vi "Make Default FFmeter settings.vi"() -> (3 "FFmeter settings":T1={"AC Source"={"AC Source type"=enum."Agilent 331xxA to 332xxA", "awg lib session"={"type"=enum."Agilent 331xxA to 332xxA", "VISA"="", "enable 10MHz ref"=FALSE, "cmi ckd2"={"VISA"="", "clock source"=enum."Auto", "manual ref clk"=FALSE, "ref clock [Hz]"=0.0, "div mode"=enum."Set divisor directly"}, "cmi sync v3"={"VISA"="", "baud rate [bd/s]"=115200, "source"=enum."Auto", "hv range"=enum."1kV", "fsrc is fixed"=FALSE, "fsrc [Hz]"=10000000.0, "freq integ [s]"=1.0, "freq filter"=5, "trig level"=enum."TTL 5V", "chn1 mode"=enum."Source divider", "chn1 level"=enum."Positive 5V", "chn2 mode"=enum."Source divider", "chn2 level"=enum."Positive 5V", "chn2 div"=1, "chn3 mode"=enum."Chn 1 Active", "chn3 level"=enum."Positive 5V", "chn1 div entry"=enum."Calculate nearest divisor from measured fx", "chn1 dev limit [%]"=1.0, "chn1 check dev"=FALSE}, "trigger"={"source"=enum."Immediate", "level [V]"=0.0, "coupling"=enum."DC", "slope"=enum."POS"}, "HMF2500 cfg"={"Baud Rate"=9600, "Parity"=0, "Data Bits"=8, "Flow Control"=4}}, "DAQmx Device Name"="PXI2Slot6"}, "TWM pipe"="\\\\.\\pipe\\TWM:server", "Measurement status ref"=refnum, "TWM Status ref"=refnum, "Abort ref"=refnum, "AC Source  status ref"=refnum, "DC meter"={"DC meter type"=enum."H/A/K 3458", "DC meter VISA"="", "NPLC"=10.0}, "Measurement properties"={"Measurement frequencies (Hz)"=[1000.0], "Sampling frequency (Hz)"=500000.0, "Signal amplitude (V)"=4.5, "AC-DC settle time (s)"=20.0, "Record length (multiples of period)"=[1000.0, 10000.0, 1000.0], "Measurement template file"=path "", "Row of START keyword"=1, "Row of STOP keyword"=0}} {"Measurement properties"."Record length (multiples of period)" format="%#_3p"; "Measurement properties"."Sampling frequency (Hz)" format="%#_3p"; "Measurement properties"."Measurement frequencies (Hz)" format="%#_3p"; "AC Source"."awg lib session"."HMF2500 cfg"."Flow Control" items=["None", "XON/XOFF", "RTS/CTS", "XON/XOFF & RTS/CTS", "DTR/DSR", "XON/XOFF & DTR/DSR"]; "AC Source"."awg lib session"."HMF2500 cfg"."Data Bits" items=["7"=7, "8"=8]; "AC Source"."awg lib session"."HMF2500 cfg"."Parity" items=["None", "Odd", "Even", "Mark", "Space"]; "AC Source"."awg lib session"."HMF2500 cfg"."Baud Rate" items=["300"=300, "600"=600, "1200"=1200, "2400"=2400, "4800"=4800, "9600"=9600, "19200"=19200]; "AC Source"."awg lib session"."cmi sync v3"."chn2 div" min=1 max=100000000 step=1; "AC Source"."awg lib session"."cmi sync v3"."fsrc [Hz]" format="%_8p"})   [LabVIEW 2020]
doc: "Returns QPS set to default values."
uses:
  GUI/Type definitions/FFmeter settings.ctl
  General AC source/Type definitions/AC Source.ctl
  General AC source/Type definitions/AC Source type.ctl
  external libraries/AWG/AWG Session.ctl
  external libraries/AWG/AWG Type.ctl
  external libraries/AWG/CMI Clock Divider v2/CMI ckd2 Session.ctl
  external libraries/AWG/CMI Clock Divider v2/CMI ckd2 Source Mode.ctl
  external libraries/AWG/CMI Clock Divider v2/CMI ckd2 Divisor Mode.ctl
  external libraries/AWG/CMI Sync V3/CMI Sync V3 session.ctl
  external libraries/AWG/CMI Sync V3/Configure/CMI Sync V3 Reference Clock Source.ctl
  external libraries/AWG/CMI Sync V3/Configure/CMI Sync V3 HV input Range.ctl
  external libraries/AWG/CMI Sync V3/Configure/CMI Sync V3 Trigger Input Level.ctl
  external libraries/AWG/CMI Sync V3/Configure/CMI Sync V3 Channel 1 Mode.ctl
  external libraries/AWG/CMI Sync V3/Configure/CMI Sync V3 Channel Output Levels.ctl
  external libraries/AWG/CMI Sync V3/Configure/CMI Sync V3 Channel 2 Mode.ctl
  external libraries/AWG/CMI Sync V3/Configure/CMI Sync V3 Channel 3 Mode.ctl
  external libraries/AWG/CMI Sync V3/Configure/CMI Sync V3 Channel 1 Divisor Entry Mode.ctl
  external libraries/externals needed for AWG/ADC Trig Config.ctl
  external libraries/externals needed for AWG/ADC Trig Mode Source.ctl
  external libraries/externals needed for AWG/ADC Trig Coupling.ctl
  external libraries/externals needed for AWG/ADC Trig Slope.ctl
  external libraries/AWG/RaS HMF2500/HMF2500 Config.ctl
  General DC meter/Type definitions/DC meter.ctl
  General DC meter/Type definitions/DC meter type.ctl
  Measurement/Type definitions/Measuement properties.ctl
  external libraries/AWG/AWG.lvlib
  external libraries/AWG/CMI Sync V3/CMI Sync Unit V3.lvlib
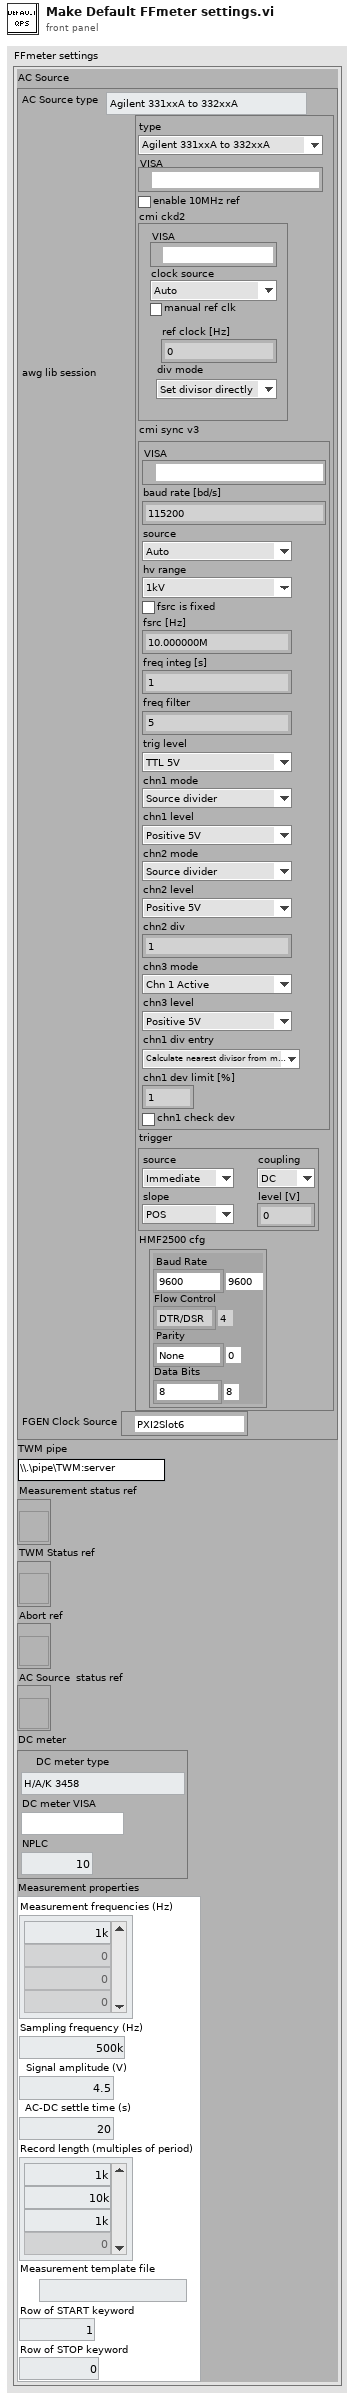
[diagram p1: front panel]
types:
  T1 = typedef "FFmeter settings.ctl" = cluster{"AC Source":T2, "TWM pipe":string, "Measurement status ref":refnum<vi>, "TWM Status ref":refnum<vi>, "Abort ref":refnum<vi>, "AC Source  status ref":refnum<vi>, "DC meter":T23, "Measurement properties":T25}
  T2 = typedef "AC Source.ctl" = cluster{"AC Source type":T3, "awg lib session":T4, "DAQmx Device Name":tag}
  T3 = typedef "AC Source type.ctl" = enum16{"Agilent 331xxA to 332xxA", "Agilent 335xxA to 336xxA", "Tektronix AFG3101C", "R&S HMF25xx", "CMI Clock Divider v2", "CMI Sync Unit V3", "NI DAQ", "Fluke 5XXX calibrator", "dummy"}
  T4 = typedef "AWG.lvlib/AWG Session.ctl" = cluster{"type":T5, "VISA":refnum<visa-resource-name>, "enable 10MHz ref":bool, "cmi ckd2":T6, "cmi sync v3":T9, "trigger":T18, "HMF2500 cfg":T22}
  T5 = typedef "AWG.lvlib/AWG Type.ctl" = enum16{"Agilent 331xxA to 332xxA", "Agilent 335xxA to 336xxA", "Tektronix AFG3101C", "R&S HMF25xx", "CMI Clock Divider v2", "CMI Sync Unit V3", "dummy"}
  T6 = typedef "AWG.lvlib/CMI ckd2 Session.ctl" = cluster{"VISA":refnum<visa-resource-name>, "clock source":T7, "manual ref clk":bool, "ref clock [Hz]":dbl, "div mode":T8}
  T7 = typedef "AWG.lvlib/CMI ckd2 Source Mode.ctl" = enum16{"Auto", "LF clock", "HF clock", "Internal"}
  T8 = typedef "AWG.lvlib/CMI ckd2 Divisor Mode.ctl" = enum16{"Set divisor directly", "Set divisor by frequency"}
  T9 = typedef "AWG.lvlib/CMI Sync Unit V3.lvlib/CMI Sync V3 session.ctl" = cluster{"VISA":refnum<visa-resource-name>, "baud rate [bd/s]":i32, "source":T10, "hv range":T11, "fsrc is fixed":bool, "fsrc [Hz]":dbl, "freq integ [s]":dbl, "freq filter":i32, "trig level":T12, "chn1 mode":T13, "chn1 level":T14, "chn2 mode":T15, "chn2 level":T14, "chn2 div":i32, "chn3 mode":T16, "chn3 level":T14, "chn1 div entry":T17, "chn1 dev limit [%]":dbl, "chn1 check dev":bool}
  T10 = typedef "AWG.lvlib/CMI Sync Unit V3.lvlib/CMI Sync V3 Reference Clock Source.ctl" = enum16{"Auto", "Internal", "Logic", "Sine", "HV"}
  T11 = typedef "AWG.lvlib/CMI Sync Unit V3.lvlib/CMI Sync V3 HV input Range.ctl" = enum16{"10V", "60V", "250V", "1kV"}
  T12 = typedef "AWG.lvlib/CMI Sync Unit V3.lvlib/CMI Sync V3 Trigger Input Level.ctl" = enum16{"LVCMOS 3V3", "TTL 5V"}
  T13 = typedef "AWG.lvlib/CMI Sync Unit V3.lvlib/CMI Sync V3 Channel 1 Mode.ctl" = enum16{"Source divider", "DDS absolute", "DDS ratio", "DDS ratio M/N"}
  T14 = typedef "AWG.lvlib/CMI Sync Unit V3.lvlib/CMI Sync V3 Channel Output Levels.ctl" = enum16{"Positive 3V3", "Negative 3V3", "Positive 5V", "Negative 5V"}
  T15 = typedef "AWG.lvlib/CMI Sync Unit V3.lvlib/CMI Sync V3 Channel 2 Mode.ctl" = enum16{"Source divider", "Chn 1 divide"}
  T16 = typedef "AWG.lvlib/CMI Sync Unit V3.lvlib/CMI Sync V3 Channel 3 Mode.ctl" = enum16{"Chn 1 Active", "Chn 2 Active", "Chn 1 Trigger", "Chn 2 Trigger", "Gate", "PPS", "10MHz"}
  T17 = typedef "AWG.lvlib/CMI Sync Unit V3.lvlib/CMI Sync V3 Channel 1 Divisor Entry Mode.ctl" = enum16{"Set divisor directly", "Calculate nearest divisor from measured fx"}
  T18 = typedef "ADC Trig Config.ctl" = cluster{"source":T19, "level [V]":dbl, "coupling":T20, "slope":T21}
  T19 = typedef "ADC Trig Mode Source.ctl" = enum16{"Immediate", "External", "Level"}
  T20 = typedef "ADC Trig Coupling.ctl" = enum16{"DC", "AC"}
  T21 = typedef "ADC Trig Slope.ctl" = enum16{"POS", "NEG"}
  T22 = typedef "AWG.lvlib/HMF2500 Config.ctl" = cluster{"Baud Rate":u32, "Parity":u16, "Data Bits":u16, "Flow Control":u16}
  T23 = typedef "DC meter.ctl" = cluster{"DC meter type":T24, "DC meter VISA":refnum<visa-resource-name>, "NPLC":dbl}
  T24 = typedef "DC meter type.ctl" = enum16{"H/A/K 3458", "FLuke 8508A", "dummy"}
  T25 = typedef "Measuement properties.ctl" = cluster{"Measurement frequencies (Hz)":dbl[], "Sampling frequency (Hz)":dbl, "Signal amplitude (V)":dbl, "AC-DC settle time (s)":dbl, "Record length (multiples of period)":dbl[], "Measurement template file":path, "Row of START keyword":i32, "Row of STOP keyword":i32}
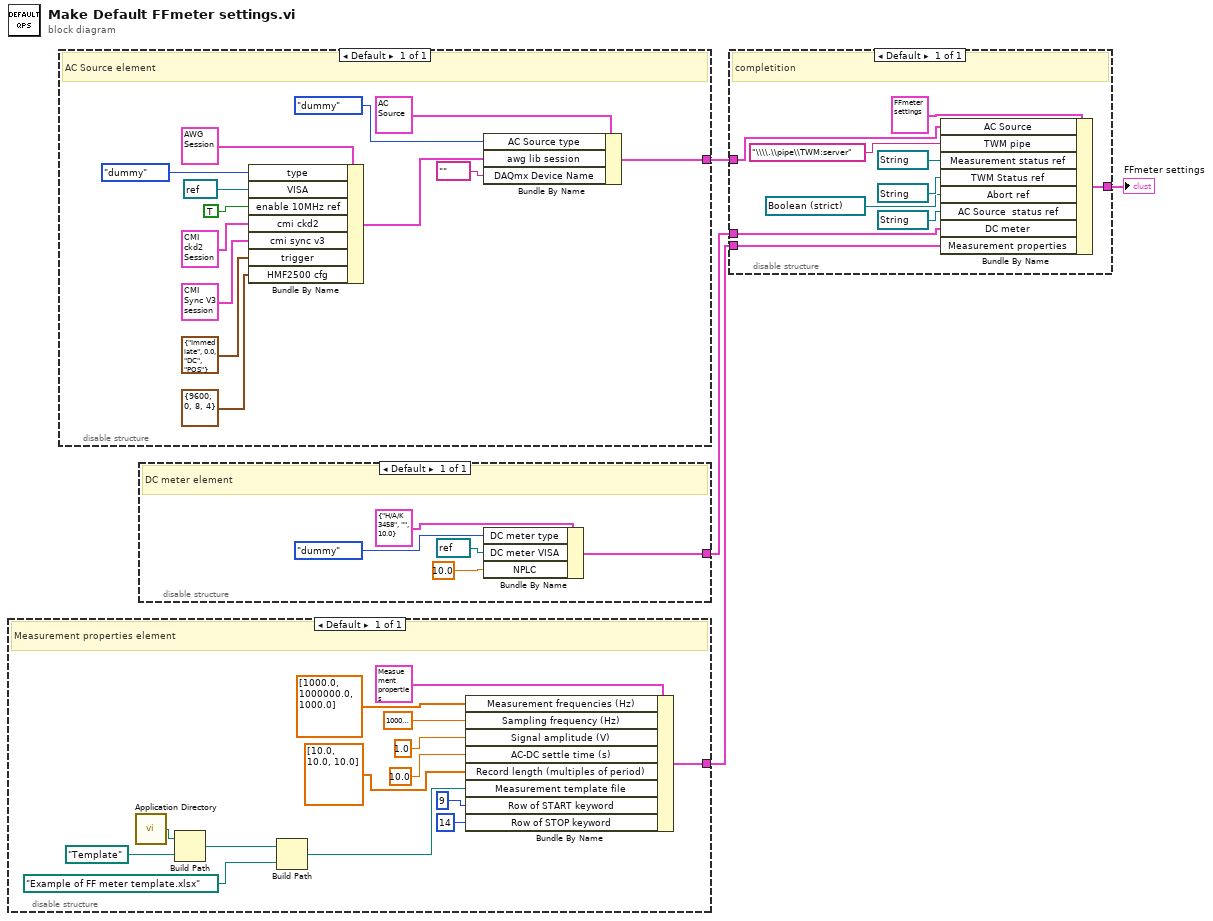
[diagram p0: block diagram]
diagram:
  n1 = disable-structure shown="Default" {
    disable-tunnel: [w17] -> w1
    frame Enabled {
      # "Measurement properties element"
      n2 = call <vilib>:"Application Directory.vi"() -> ("Application Directory"=w5:path)
      n3 = Build Path(base path=w5, name or relative path=path "Template") -> (appended path=w8:path)
      n4 = Build Path(base path=w8, name or relative path=path "Example of FF meter template.xlsx") -> (appended path=w6:path)
      n5 = Bundle By Name(cluster=T25 {"Measurement frequencies (Hz)"=[1000.0, 10000.0, 1000.0], "Sampling frequency (Hz)"=500000.0, "Signal amplitude (V)"=4.5, "AC-DC settle time (s)"=20.0, "Record length (multiples of period)"=[1000.0, 10000.0, 1000.0], "Measurement template file"=path "", "Row of START keyword"=0, "Row of STOP keyword"=0} ("Measurement properties"), "Measurement frequencies (Hz)"=dbl[] [1000.0, 1000000.0, 1000.0], "Sampling frequency (Hz)"=10000000.0, "Signal amplitude (V)"=1.0, "AC-DC settle time (s)"=10.0, "Record length (multiples of period)"=dbl[] [10.0, 10.0, 10.0], "Measurement template file"=w6, "Row of START keyword"=9, "Row of STOP keyword"=14) -> (w17:T25)
    }
  }
  n6 = disable-structure shown="Default" {
    disable-tunnel: [w22] -> w4
    frame Enabled {
      # "AC Source element"
      n7 = Bundle By Name(cluster=T4 {"type"=enum."Agilent 331xxA to 332xxA", "VISA"="", "enable 10MHz ref"=FALSE, "cmi ckd2"={"VISA"="", "clock source"=enum."Auto", "manual ref clk"=FALSE, "ref clock [Hz]"=0.0, "div mode"=enum."Set divisor directly"}, "cmi sync v3"={"VISA"="", "baud rate [bd/s]"=115200, "source"=enum."Auto", "hv range"=enum."1kV", "fsrc is fixed"=FALSE, "fsrc [Hz]"=10000000.0, "freq integ [s]"=1.0, "freq filter"=5, "trig level"=enum."TTL 5V", "chn1 mode"=enum."Source divider", "chn1 level"=enum."Positive 5V", "chn2 mode"=enum."Source divider", "chn2 level"=enum."Positive 5V", "chn2 div"=1, "chn3 mode"=enum."Chn 1 Active", "chn3 level"=enum."Positive 5V", "chn1 div entry"=enum."Calculate nearest divisor from measured fx", "chn1 dev limit [%]"=1.0, "chn1 check dev"=FALSE}, "trigger"={"source"=enum."Immediate", "level [V]"=0.0, "coupling"=enum."DC", "slope"=enum."POS"}, "HMF2500 cfg"={"Baud Rate"=9600, "Parity"=0, "Data Bits"=8, "Flow Control"=4}} ("awg session"), "type"=AWG_Type."dummy", "VISA"=refnum<visa-resource-name> refnum, "enable 10MHz ref"=TRUE, "cmi ckd2"=T6 {"VISA"="", "clock source"=enum."Auto", "manual ref clk"=FALSE, "ref clock [Hz]"=0.0, "div mode"=enum."Set divisor directly"}, "cmi sync v3"=T9 {"VISA"="", "baud rate [bd/s]"=115200, "source"=enum."Auto", "hv range"=enum."1kV", "fsrc is fixed"=FALSE, "fsrc [Hz]"=10000000.0, "freq integ [s]"=1.0, "freq filter"=5, "trig level"=enum."TTL 5V", "chn1 mode"=enum."Source divider", "chn1 level"=enum."Positive 5V", "chn2 mode"=enum."Source divider", "chn2 level"=enum."Positive 5V", "chn2 div"=1, "chn3 mode"=enum."Chn 1 Active", "chn3 level"=enum."Positive 5V", "chn1 div entry"=enum."Calculate nearest divisor from measured fx", "chn1 dev limit [%]"=1.0, "chn1 check dev"=FALSE}, "trigger"=T18 {"source"=enum."Immediate", "level [V]"=0.0, "coupling"=enum."DC", "slope"=enum."POS"}, "HMF2500 cfg"=T22 {"Baud Rate"=9600, "Parity"=0, "Data Bits"=8, "Flow Control"=4}) -> (w23:T4)
      n8 = Bundle By Name(cluster=T2 {"AC Source type"=enum."Agilent 331xxA to 332xxA", "awg lib session"={"type"=enum."Agilent 331xxA to 332xxA", "VISA"="", "enable 10MHz ref"=FALSE, "cmi ckd2"={"VISA"="", "clock source"=enum."Auto", "manual ref clk"=FALSE, "ref clock [Hz]"=0.0, "div mode"=enum."Set divisor directly"}, "cmi sync v3"={"VISA"="", "baud rate [bd/s]"=115200, "source"=enum."Auto", "hv range"=enum."1kV", "fsrc is fixed"=FALSE, "fsrc [Hz]"=10000000.0, "freq integ [s]"=1.0, "freq filter"=5, "trig level"=enum."TTL 5V", "chn1 mode"=enum."Source divider", "chn1 level"=enum."Positive 5V", "chn2 mode"=enum."Source divider", "chn2 level"=enum."Positive 5V", "chn2 div"=1, "chn3 mode"=enum."Chn 1 Active", "chn3 level"=enum."Positive 5V", "chn1 div entry"=enum."Calculate nearest divisor from measured fx", "chn1 dev limit [%]"=1.0, "chn1 check dev"=FALSE}, "trigger"={"source"=enum."Immediate", "level [V]"=0.0, "coupling"=enum."DC", "slope"=enum."POS"}, "HMF2500 cfg"={"Baud Rate"=9600, "Parity"=0, "Data Bits"=8, "Flow Control"=4}}, "DAQmx Device Name"="PXI2Slot6"} ("AC Source"), "AC Source type"=AC_Source_type."dummy" ("AWG type"), "awg lib session"=w23, "DAQmx Device Name"=tag "") -> (w22:T2)
    }
  }
  n9 = disable-structure shown="Default" {
    disable-tunnel: [w35] -> w2
    frame Enabled {
      # "DC meter element"
      n10 = Bundle By Name(cluster=T23 {"DC meter type"=enum."H/A/K 3458", "DC meter VISA"="", "NPLC"=10.0} ("DC meter"), "DC meter type"=DC_meter_type."dummy", "DC meter VISA"=refnum<visa-resource-name> refnum, "NPLC"=10.0) -> (w35:T23)
    }
  }
  n11 = disable-structure shown="Default" {
    disable-tunnel: [w46] -> w3
    disable-tunnel: w4 -> [w43]
    disable-tunnel: w2 -> [w38]
    disable-tunnel: w1 -> [w37]
    frame Enabled {
      # "completition"
      n12 = Bundle By Name(cluster=T1 {"AC Source"={"AC Source type"=enum."Agilent 331xxA to 332xxA", "awg lib session"={"type"=enum."Agilent 331xxA to 332xxA", "VISA"="", "enable 10MHz ref"=FALSE, "cmi ckd2"={"VISA"="", "clock source"=enum."Auto", "manual ref clk"=FALSE, "ref clock [Hz]"=0.0, "div mode"=enum."Set divisor directly"}, "cmi sync v3"={"VISA"="", "baud rate [bd/s]"=115200, "source"=enum."Auto", "hv range"=enum."1kV", "fsrc is fixed"=FALSE, "fsrc [Hz]"=10000000.0, "freq integ [s]"=1.0, "freq filter"=5, "trig level"=enum."TTL 5V", "chn1 mode"=enum."Source divider", "chn1 level"=enum."Positive 5V", "chn2 mode"=enum."Source divider", "chn2 level"=enum."Positive 5V", "chn2 div"=1, "chn3 mode"=enum."Chn 1 Active", "chn3 level"=enum."Positive 5V", "chn1 div entry"=enum."Calculate nearest divisor from measured fx", "chn1 dev limit [%]"=1.0, "chn1 check dev"=FALSE}, "trigger"={"source"=enum."Immediate", "level [V]"=0.0, "coupling"=enum."DC", "slope"=enum."POS"}, "HMF2500 cfg"={"Baud Rate"=9600, "Parity"=0, "Data Bits"=8, "Flow Control"=4}}, "DAQmx Device Name"="PXI2Slot6"}, "TWM pipe"="\\\\.\\pipe\\TWM:server", "Measurement status ref"=refnum, "TWM Status ref"=refnum, "Abort ref"=refnum, "AC Source  status ref"=refnum, "DC meter"={"DC meter type"=enum."H/A/K 3458", "DC meter VISA"="", "NPLC"=10.0}, "Measurement properties"={"Measurement frequencies (Hz)"=[1000.0], "Sampling frequency (Hz)"=500000.0, "Signal amplitude (V)"=4.5, "AC-DC settle time (s)"=20.0, "Record length (multiples of period)"=[1000.0, 10000.0, 1000.0], "Measurement template file"=path "", "Row of START keyword"=1, "Row of STOP keyword"=0}} ("FFmeter settings"), "AC Source"=w43, "TWM pipe"="\\\\.\\pipe\\TWM:server" ("TWM pipe name"), "Measurement status ref"=refnum<vi> refnum, "TWM Status ref"=refnum<vi> refnum, "Abort ref"=refnum<vi> refnum, "AC Source  status ref"=refnum<vi> refnum, "DC meter"=w38, "Measurement properties"=w37) -> (w46:T1)
    }
  }
  "FFmeter settings" <- w3
